vi "2023 Read Arm to Phi Spreadsheet.vi"(2 "error in":errorcluster, 3 "output array 2":dbl[](array[numeric]), 4 "Arm Angle":dbl=22.5) -> (0 "error out":errorcluster, 1 "y value":dbl)   [LabVIEW 2020]
uses:
  2023ArmReachSpreadsheetGlobal.vi
panel:
  out "wristAngle":dbl
  out "X1":dbl
  out "X2":dbl
  out "Y2":dbl
  out "CeilingRowJ":i32
  out "FloorRowJ":i32
  out "CeilingRowI":i32
  out "Y1":dbl
  out "FloorRowI":i32
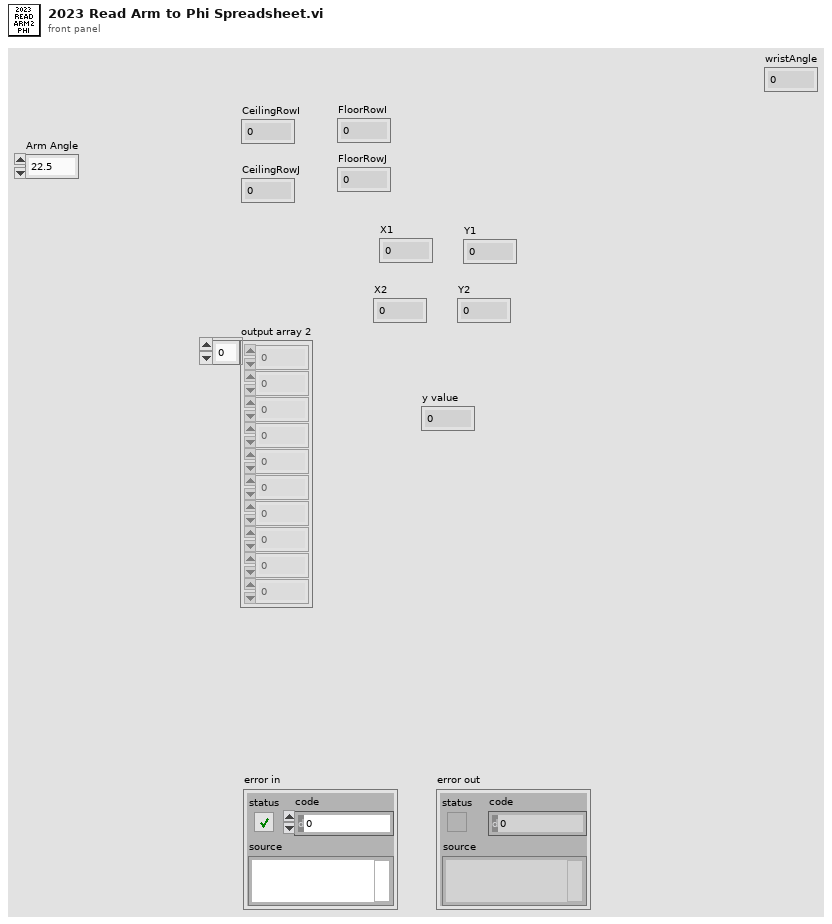
[diagram p1: front panel]
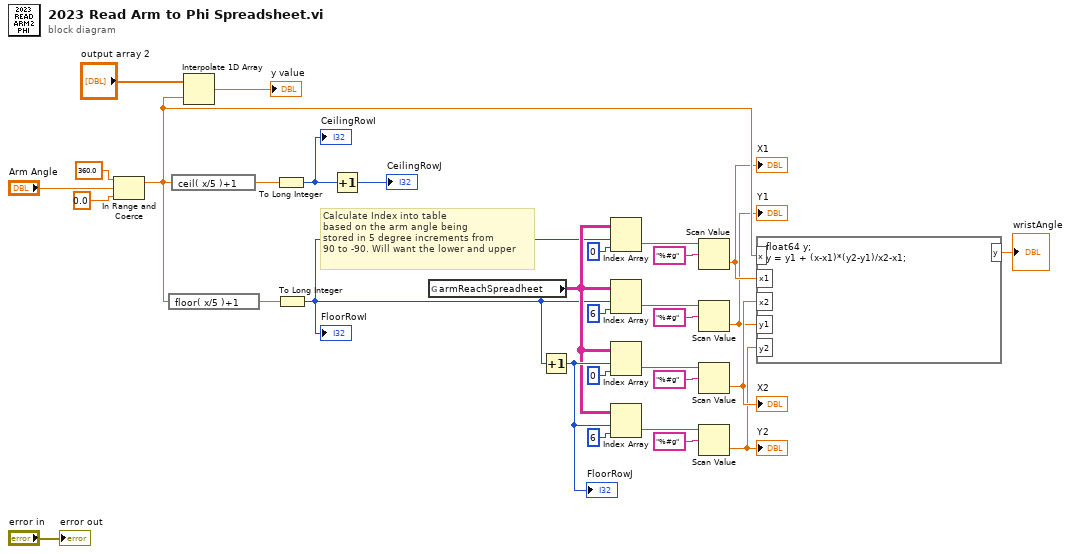
[diagram p0: block diagram]
diagram:
  # "Calculate Index into table\nbased on the arm angle being\nstored in 5 degree increments from\n90 to -90. Will want the lower and upper"
  n1 = In Range and Coerce(upper limit=360.0, x="Arm Angle", lower limit=0.0) -> (coerced(x)=w6:dbl)  [unwired: 1 out]
  n2 = expression code="floor( x/5 )+1"(w6) -> (w27:dbl)
  n3 = expression code="ceil( x/5 )+1"(w6) -> (w21:dbl)
  n4 = Interpolate 1D Array(1:w6, 2:"output array 2") -> (0:→"y value":dbl)
  n5 = To Long Integer(number=w21) -> (32bit integer=w20:i32)
  "CeilingRowI" <- w20
  n6 = To Long Integer(number=w27) -> (32bit integer=w10:i32)
  "FloorRowI" <- w10
  n7 = Increment(x=w20) -> (x+1=→"CeilingRowJ":i32)
  n8 = global read "2023ArmReachSpreadsheetGlobal.vi" "armReachSpreadheet"() -> (w11:string[][])
  n9 = Increment(x=w10) -> (x+1=w17:i32)
  "FloorRowJ" <- w17
  n10 = Index Array(array=w11, index (row)=w10, index (col)=0 ("disabled index (col)")) -> (element=w7:string)
  n11 = Index Array(array=w11, index (row)=w10, index (col)=6 ("disabled index (col)")) -> (element=w24:string)
  n12 = Index Array(array=w11, index (row)=w17, index (col)=0) -> (element=w12:string)
  n13 = Index Array(array=w11, index (row)=w17, index (col)=6) -> (element=w14:string)
  n14 = Scan Value(string=w7, format string="%#g") -> (value=w5:dbl)  [unwired: 1 in, 1 out]
  "X1" <- w5
  n15 = Scan Value(string=w24, format string="%#g") -> (value=w3:dbl)  [unwired: 1 in, 1 out]
  "Y1" <- w3
  n16 = Scan Value(string=w12, format string="%#g") -> (value=w4:dbl)  [unwired: 1 in, 1 out]
  "X2" <- w4
  n17 = Scan Value(string=w14, format string="%#g") -> (value=w2:dbl)  [unwired: 1 in, 1 out]
  "Y2" <- w2
  n18 = formula code="float64 y;\ny = y1 + (x-x1)*(y2-y1)/x2-x1;"("x"=w6, "x1"=w5, "x2"=w4, "y1"=w3, "y2"=w2) -> ("y"=→"wristAngle":dbl)
  "error out" <- "error in"
